vi "Noise Statistics.vi"() -> ()   [LabVIEW 2023]
doc: "Uses the various statistics VIs to generate common descriptive statistics quantities. This example determines the following statistics on Gaussian or uniform noise: standard deviation, mean, variance, mode, skewness, kurtosis, and the discrete histogram."
uses:
  <vilib>/gmath/statdist.llb/Normal Random.vi
  <vilib>/gmath/statdist.llb/Uniform Random.vi
  <vilib>/gmath/statdist.llb/Laplace Random.vi
  <vilib>/gmath/statdist.llb/Triangular Random.vi
  <vilib>/gmath/statdist.llb/Beta Random.vi
  <vilib>/Analysis/baseanly.llb/Unimode.vi
  <vilib>/Analysis/NI_AALBase.lvlib
  <vilib>/gmath/NI_Gmath.lvlib
panel:
  in  "Instructions":string="Overview: Uses various Probability & Statistics VIs to generate common descriptive statistics quantities.\nRequirements: LabVIEW Full Development System\nInstructions: \n1. Run the VI and choose a Distribution that you would like to study. Note that if you specify a Seed larger than zero, it will keep the same number sequence. If you specify a Seed of '-1', a random seed value will be used.\n2. Change the properties of the generated signal and verify how it affects the statistics measure.\n3. Change the Histogram Interval to verify how it changes the number of bars on the histogram.\n4. Click Stop to stop the VI."
  out "Median":dbl format="%0.2f"
  in  "Parameter":dbl(slide)=2.0 scale=0.1..100.0
  in  "Skew":dbl(slide) scale=-10.0..10.0
  in  "Spreading":dbl(slide)=10.0 scale=3.0..20.0
  in  "Average":dbl(slide) scale=-5.0..5.0
  in  "Stop":bool
  out "Normal Probability Density Function":cluster{"X Values":dbl[], dbl[]}(graph)
  out "Signal Generated":dbl[](graph)
  in  "Seed":i32=2
  in  "Distribution":u16(ring) items=["Normal", "Uniform", "Laplace (Gumbel)", "Triangular", "Beta"]
  out "Mode":dbl format="%0.2f"
  out "Kurtosis":dbl format="%0.2f"
  out "Skewness":dbl format="%0.2f"
  out "Variance":dbl format="%0.2f"
  out "Standard Deviation":dbl format="%0.2f"
  out "Mean":dbl format="%0.2f"
  in  "Histogram Interval":i32(slide)=50 scale=3.0..100.0
  # "Measures of Mean"
  # "Measures of Spread"
  # "Shape Parameters"
  # "Kurtosis larger than 3 indicates a sharper peak than a Normal Distribution."
  # "Skewness less than zero indicates that the peak goes to the right."
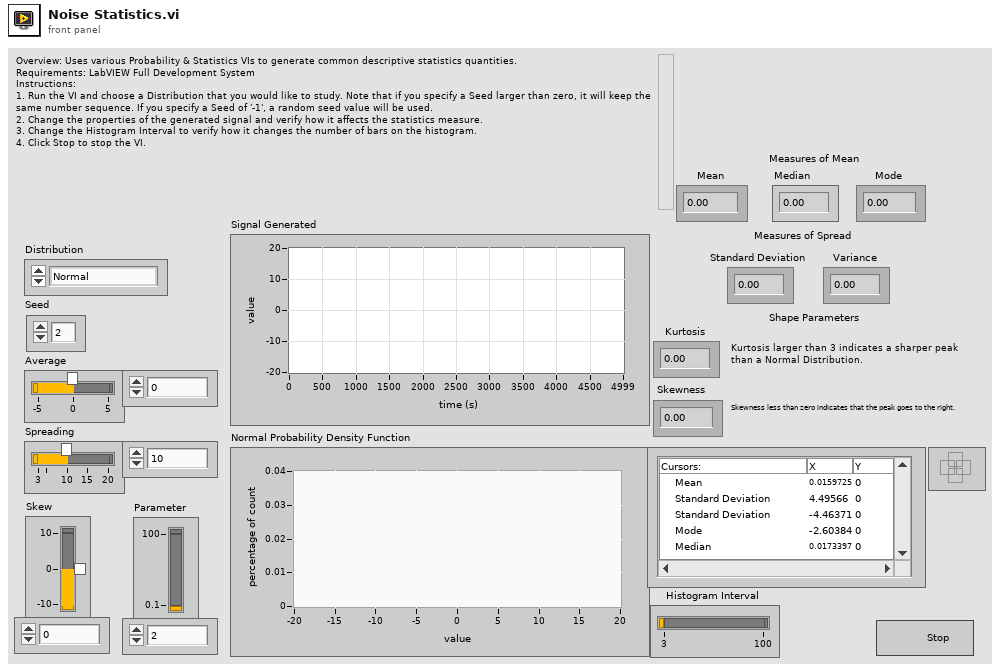
[diagram p1: front panel]
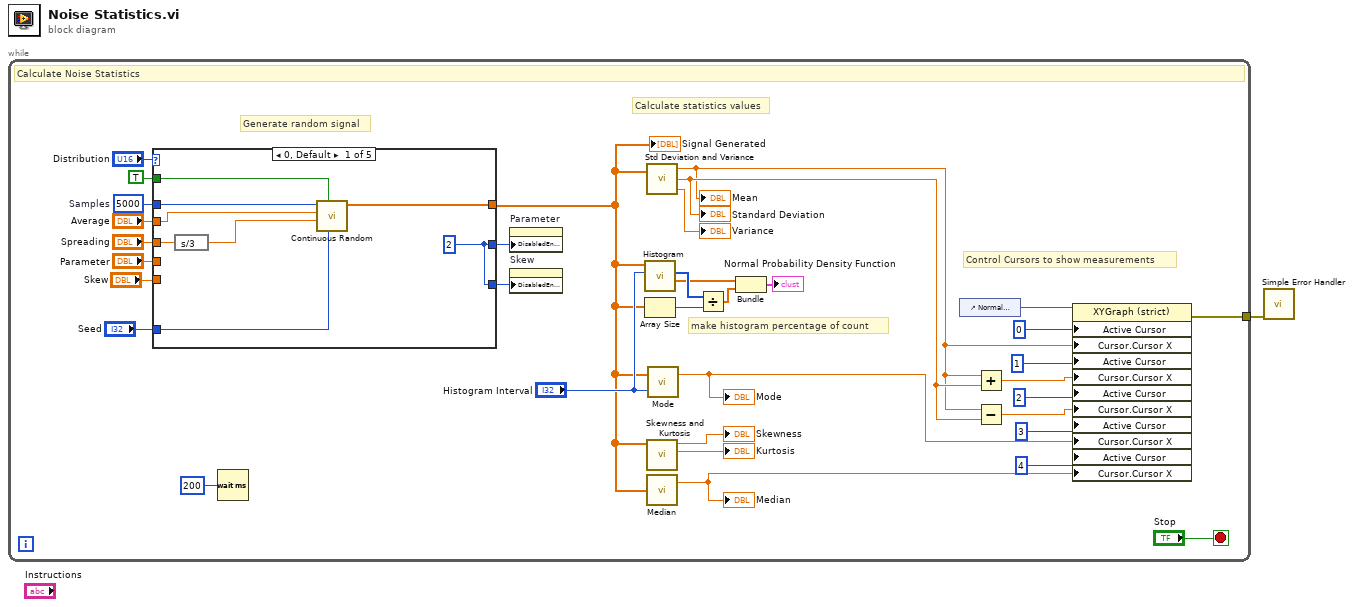
[diagram p0: block diagram]
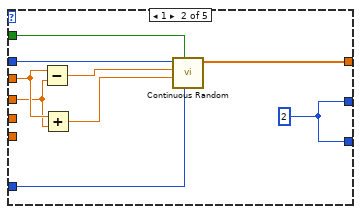
[diagram p2: hidden frame]
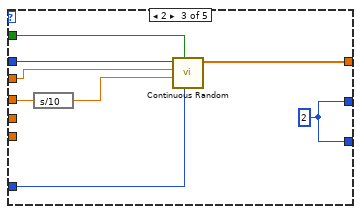
[diagram p3: hidden frame]
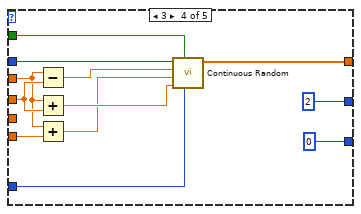
[diagram p4: hidden frame]
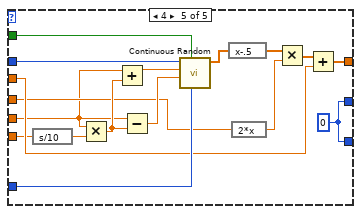
[diagram p5: hidden frame]
diagram:
  n1 = while {
    tunnel: [w2] -> w1
    stop <- "Stop" stop-if-true
    w9 = 5000  # Samples
    # "Control Cursors to show measurements"
    # "Generate random signal"
    # "make histogram percentage of count"
    # "Calculate statistics values"
    # "Calculate Noise Statistics"
    n2 = case shown="0, Default" "Distribution" {
      tunnel: [w44 w53 w61 w73 w87] -> w5
      tunnel: w9 -> [w43 w52 w60 w72 w90]
      tunnel: "Seed" -> [w42 w51 w59 w71 w89]
      tunnel: TRUE ("reset") -> [w41 w50 w58 w70 w88]
      tunnel: "Average" -> [w40 w47 w57 w66 w86]
      tunnel: "Spreading" -> [w38 w46 w55 w68 w78]
      tunnel: "Skew" -> [_ _ _ w65 w83]
      tunnel: "Parameter" -> [_ _ _ _ w75]
      tunnel: [w39 w45 w56 2 w84] -> w4
      tunnel: [w39 w45 w56 0 w84] -> w3
      frame 0, Default {
        w39 = 2
        n3 = expression code="s/3"(w38) -> (w37:dbl)
        n4 = call-poly <vilib>:"Continuous Random.vi"("seed"=w42, "reset"=w41, "std"=w37, "mean"=w40, "samples"=w43) -> ("normal random data"=w44:dbl[])  [unwired: 5 in, 1 out]
      }
      frame 1 {
        w45 = 2
        n5 = Subtract(x=w47, y=w46) -> (x-y=w48:dbl)
        n6 = Add(x=w47, y=w46) -> (x+y=w49:dbl)
        n7 = call-poly <vilib>:"Continuous Random.vi"("seed"=w51, "reset"=w50, "xmax"=w49, "xmin"=w48, "samples"=w52) -> ("uniform random data"=w53:dbl[])  [unwired: 5 in, 1 out]
      }
      frame 2 {
        w56 = 2
        n8 = expression code="s/10"(w55) -> (w54:dbl)
        n9 = call-poly <vilib>:"Continuous Random.vi"("seed"=w59, "reset"=w58, "b"=w54, "a"=w57, "samples"=w60) -> ("Laplace random numbers"=w61:dbl[])  [unwired: 5 in, 1 out]
      }
      frame 3 {
        n10 = Subtract(x=w66, y=w68) -> (x-y=w69:dbl)
        n11 = Add(x=w66, y=w68) -> (x+y=w67:dbl)
        n12 = Add(x=w66, y=w65) -> (x+y=w64:dbl)
        n13 = call-poly <vilib>:"Continuous Random.vi"("seed"=w71, "reset"=w70, "xmax"=w67, "xmode"=w64, "xmin"=w69, "samples"=w72) -> ("triangular random data"=w73:dbl[])  [unwired: 4 in, 1 out]
      }
      frame 4 {
        w84 = 0
        n14 = expression code="s/10"(w83) -> (w82:dbl)
        n15 = Multiply(x=w75, y=w82) -> (x*y=w81:dbl)
        n16 = Add(x=w75, y=w81) -> (x+y=w80:dbl)
        n17 = Subtract(x=w75, y=w81) -> (x-y=w79:dbl)
        n18 = call-poly <vilib>:"Continuous Random.vi"("seed"=w89, "reset"=w88, "b"=w79, "a"=w80, "samples"=w90) -> ("beta random data"=w74:dbl[])  [unwired: 5 in, 1 out]
        n19 = expression code="x-.5"(w74) -> (w76:dbl[])
        n20 = expression code="2*x"(w78) -> (w77:dbl)
        n21 = Multiply(x=w76, y=w77) -> (x*y=w85:dbl[])
        n22 = Add(x=w85, y=w86) -> (x+y=w87:dbl[])
      }
    }
    "Signal Generated" <- w5
    n23 = Wait (ms)(milliseconds to wait=u32 200) -> ()  [unwired: 1 out]
    n24 = property on="Parameter" class="Slide (strict)"("DisabledEnum"=w4) -> ()  [unwired: 2 in, 2 out]
    n25 = property on="Skew" class="Slide (strict)"("DisabledEnum"=w3) -> ()  [unwired: 2 in, 2 out]
    n26 = call <vilib>:"Histogram.vi"("intervals"="Histogram Interval", "X"=w5) -> ("X Values"=w8:dbl[], "Histogram: h(x)"=w11:i32[])  [unwired: 6 in, 2 out]
    n27 = Array Size(array=w5) -> (size(s)=w6:i32)
    n28 = call <vilib>:"Std Deviation and Variance.vi"("X"=w5) -> ("mean"=w17:dbl, "standard deviation"=w21:dbl, "variance"=→"Variance":dbl)  [unwired: 1 in]
    "Mean" <- w17
    "Standard Deviation" <- w21
    n29 = call <vilib>:"Skewness and Kurtosis.vi"("X"=w5) -> ("kurtosis"=→"Kurtosis":dbl, "skewness"=→"Skewness":dbl)  [unwired: 8 in, 1 out]
    n30 = call <vilib>:"Median.vi"("X"=w5) -> ("median"=w12:dbl)  [unwired: 1 out]
    "Median" <- w12
    n31 = call-poly <vilib>:"Mode.vi"("intervals"="Histogram Interval", "X"=w5) -> ("mode"=w14:dbl)  [unwired: 1 out]
    "Mode" <- w14
    n32 = Divide(x=w11, y=w6) -> (x/y=w10:dbl[])
    n33 = Bundle("X Values"=w8, w10) -> (→"Normal Probability Density Function":cluster{"X Values":dbl[], dbl[]})  [unwired: 1 in]
    n34 = control-ref of="Normal Probability Density Function"() -> (w27:refnum<vi>)
    n35 = Add(x=w17, y=w21) -> (x+y=w30:dbl)
    n36 = Subtract(x=w17, y=w21) -> (x-y=w29:dbl)
    n37 = property on="Property Node" class="XYGraph (strict)"(reference=w27, "Active Cursor"=u32 0, "Cursor.Cursor X"=w17, "Active Cursor"=u32 1, "Cursor.Cursor X"=w30, "Active Cursor"=u32 2, "Cursor.Cursor X"=w29, "Active Cursor"=u32 3, "Cursor.Cursor X"=w14, "Active Cursor"=u32 4, "Cursor.Cursor X"=w12) -> (error out=w2:errorcluster)  [unwired: 1 in, 1 out]
  }
  n38 = call <vilib>:"Simple Error Handler.vi"("error in (no error)"=w1) -> ()  [unwired: 4 in, 5 out]
